vi "GetWaveform.vi"(8 "error in (no error)":errorcluster, 10 "Channel (1: Channel 1)":string, 11 "VISA Refnum in":refnum<visa-resource-name>) -> (0 "pt_off":dbl, 1 "Waveform":waveform(dbl), 2 "x_zero":dbl, 3 "axis labels":string)   [LabVIEW 2013]
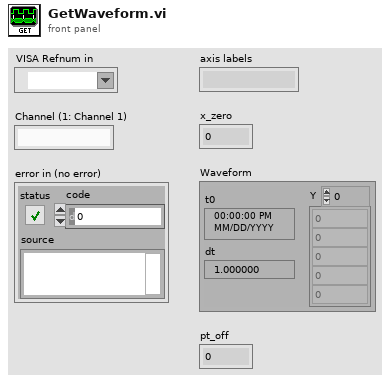
[diagram p1: front panel]
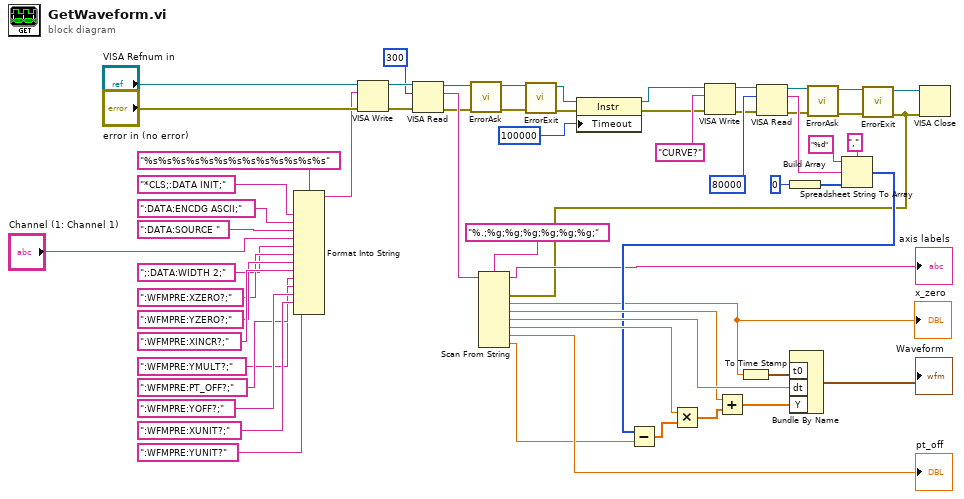
[diagram p0: block diagram]
diagram:
  n1 = Format Into String(format string="%s%s%s%s%s%s%s%s%s%s%s%s%s", "*CLS;:DATA INIT;" ("input 1"), ":DATA:ENCDG ASCII;" ("input 2"), ":DATA:SOURCE " ("input 3"), "Channel (1: Channel 1)", ";:DATA:WIDTH 2;" ("input 5"), ":WFMPRE:XZERO?;" ("input 6"), ":WFMPRE:YZERO?;" ("input 7"), ":WFMPRE:XINCR?;" ("input 8"), ":WFMPRE:YMULT?;" ("input 8"), ":WFMPRE:PT_OFF?;" ("input 8"), ":WFMPRE:YOFF?;" ("input 8"), ":WFMPRE:XUNIT?;" ("input 8"), ":WFMPRE:YUNIT?" ("input 8")) -> (resulting string=w21:string)  [unwired: 2 in, 1 out]
  n2 = VISA Write(VISA resource name="VISA Refnum in", write buffer=w21, error in (no error)="error in (no error)") -> (VISA resource name out=w26:refnum<visa-resource-name>, error out=w25:errorcluster)  [unwired: 1 out]
  n3 = VISA Read(VISA resource name=w26, byte count=u32 300, error in (no error)=w25) -> (VISA resource name out=w28:refnum<visa-resource-name>, read buffer=w59:string, error out=w29:errorcluster)  [unwired: 1 out]
  n4 = call "ErrorAsk.vi"("error in (no error)"=w29, "VISA Refnum in"=w28) -> ("error out"=w31:errorcluster, "VISA Refnum out"=w30:refnum<visa-resource-name>)  [unwired: 8 in]
  n5 = call "ErrorExit.vi"("error in (no error)"=w31, "VISA Refnum in"=w30) -> ("error out"=w4:errorcluster, "VISA Refnum out"=w5:refnum<visa-resource-name>)  [unwired: 8 in]
  n6 = property class="Instr"(reference=w5, error in=w4, "Timeout"=u32 100000 ("General Settings:Timeout Value")) -> (reference out=w3:refnum<visa-resource-name>, error out=w2:errorcluster)
  n7 = VISA Write(VISA resource name=w3, write buffer="CURVE?", error in (no error)=w2) -> (VISA resource name out=w33:refnum<visa-resource-name>, error out=w34:errorcluster)  [unwired: 1 out]
  n8 = VISA Read(VISA resource name=w33, byte count=u32 80000, error in (no error)=w34) -> (VISA resource name out=w38:refnum<visa-resource-name>, read buffer=w42:string, error out=w39:errorcluster)  [unwired: 1 out]
  n9 = Build Array(i16 0) -> (w44:i16[])
  n10 = call "ErrorAsk.vi"("error in (no error)"=w39, "VISA Refnum in"=w38) -> ("error out"=w37:errorcluster, "VISA Refnum out"=w36:refnum<visa-resource-name>)  [unwired: 8 in]
  n11 = Spreadsheet String To Array(delimiter (Tab)=",", format string="%d", spreadsheet string=w42, array type (2D Dbl)=w44) -> (array=w48:i16[])
  n12 = call "ErrorExit.vi"("error in (no error)"=w37, "VISA Refnum in"=w36) -> ("error out"=w6:errorcluster, "VISA Refnum out"=w57:refnum<visa-resource-name>)  [unwired: 8 in]
  n13 = Scan From String(format string="%.;%g;%g;%g;%g;%g;%g;", input string=w59, error in=w6) -> (remaining string=→"axis labels":string, output 1=w7:dbl, output 2=w52:dbl, output 3=w55:dbl, output 4=w50:dbl, output 5=→"pt_off":dbl, output 6=w47:dbl)  [unwired: 7 in, 2 out]
  "x_zero" <- w7
  n14 = Subtract(x=w48, y=w47) -> (x-y=w49:dbl[])
  n15 = Multiply(x=w50, y=w49) -> (x*y=w51:dbl[])
  n16 = Add(x=w52, y=w51) -> (x+y=w56:dbl[])
  n17 = To Time Stamp(1:w7) -> (0:w53:timestamp)
  n18 = Bundle By Name("t0"=w53, "dt"=w55, "Y"=w56) -> (→"Waveform":waveform(dbl))  [unwired: 1 in]
  n19 = VISA Close(VISA resource name=w57, error in (no error)=w6) -> ()  [unwired: 1 out]
